vi "avi2frame.vi"() -> ()   [LabVIEW 2010]
panel:
  in  "stop":bool
  out "Numeric":i32
  out "Number of Frames":u32
  in  "AVI Path":path
  out "Image Out":T1(plugin-control)
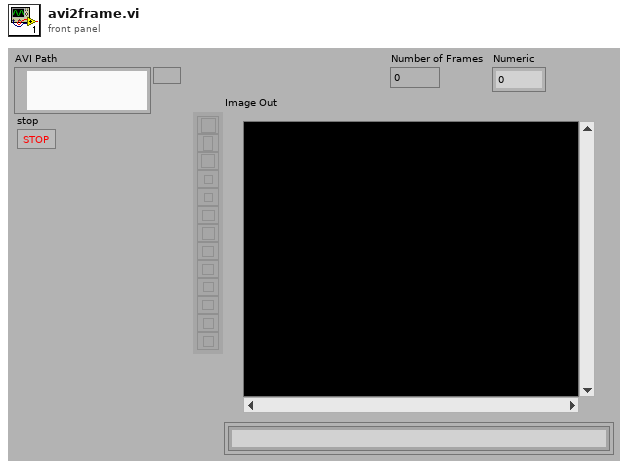
[diagram p1: front panel]
types:
  T1 = typedef "IMAQ Image.ctl" = refnum<image>
  T2 = typedef "AviRefnum.ctl" = refnum<k1>
  T3 = typedef "Image Type" = u32
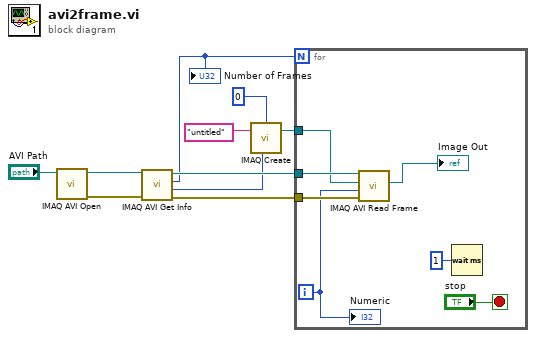
[diagram p0: block diagram]
diagram:
  n1 = call "IMAQ AVI Open"("AVI Path"="AVI Path") -> ("error out"=w7:errorcluster, "Avi Refnum"=w8:T2)  [unwired: 9 in]
  n2 = call "IMAQ AVI Get Info"("error in (no error)"=w7, "Avi Refnum"=w8) -> ("error out"=w9:errorcluster, "Image Type"=w3:T3, "Number of Frames"=w6:u32, "Avi Refnum (duplicate)"=w10:T2)  [unwired: 5 in, 1 out]
  "Number of Frames" <- w6
  n3 = call "IMAQ Create"("Border Size"=0, "Image Name"="untitled", "Image Type"=w3) -> ("New Image"=w2:T1)  [unwired: 2 in, 1 out]
  n4 = for {
    N: w6 -> [_]
    tunnel: w10 -> [w17]
    tunnel: w9 -> [w16]
    tunnel: w2 -> [w12]
    i -> [w15]
    stop <- "stop" stop-if-true
    n5 = call "IMAQ AVI Read Frame"("error in (no error)"=w16, "Frame Number"=w15, "Image"=w12, "Avi Refnum"=w17) -> ("Image Out"=→"Image Out":T1)  [unwired: 4 in, 3 out]
    n6 = Wait (ms)(milliseconds to wait=u32 1) -> ()  [unwired: 1 out]
    "Numeric" <- w15
  }
